vi "自动测试类型1统计结果.vi"   [LabVIEW 2010]
uses:
  全局量/自动测试结果.vi
  全局量/试验配置信息.vi
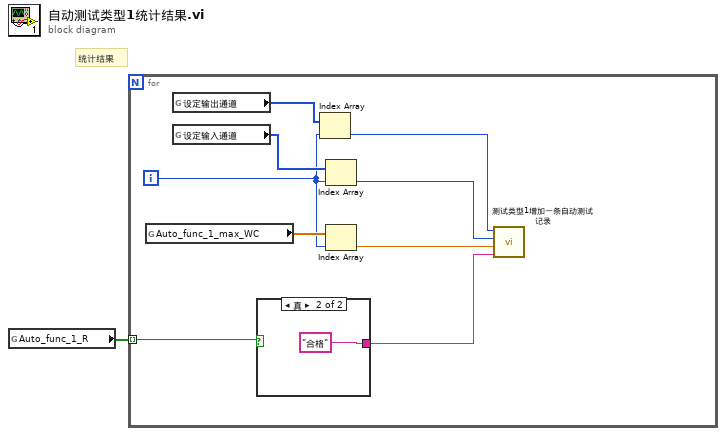
[diagram p0: block diagram]
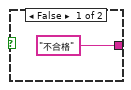
[diagram p2: hidden frame]
diagram:
  # "统计结果"
  n1 = global read "自动测试结果.vi" "Auto_func_1_R"() -> (w1:bool[])
  n2 = for {
    tunnel: w1 -> [w10] mode=indexing
    i -> [w6]
    n3 = global read "自动测试结果.vi" "Auto_func_1_max_WC"() -> (w9:dbl[])
    n4 = global read "试验配置信息.vi" "设定输出通道"() -> (w8:i32[])
    n5 = global read "试验配置信息.vi" "设定输入通道"() -> (w7:i32[])
    n6 = case shown="真" w10 {
      tunnel: ["不合格" "合格"] -> w2
      frame False {
      }
      frame True {
      }
    }
    n7 = Index Array(array=w8, index=w6) -> (element=w5:i32)
    n8 = Index Array(array=w7, index=w6) -> (element=w4:i32)
    n9 = Index Array(array=w9, index=w6) -> (element=w3:dbl)
    n10 = call "测试类型1增加一条自动测试记录.vi"("测试结果"=w2, "最大误差"=w3, "输入通道"=w4, "输出通道"=w5) -> ()  [unwired: 8 in]
  }
